vi "UserDIO and Binning Time to FPGA.vi"(8 "error in (no error)":errorcluster, 11 "FPGA VI Reference Out":refnum<k20>) -> (0 "error out":errorcluster)   [LabVIEW 2024]
uses:
  Type Definitions/DIO_Cluster.ctl
  <vilib>/Utility/error.llb/Error Cluster From Error Code.vi
  <vilib>/rvi/errors/niLvFpgaAdjustHostInterfaceError.vi
  <vilib>/rvi/interface/nirviReadWriteControl/nirviReadWriteControl.xnode
  NiFpgaLv.dll
  <vilib>/rvi/interface/Simulation/niFpgaSimulationCallBeginRW.vi
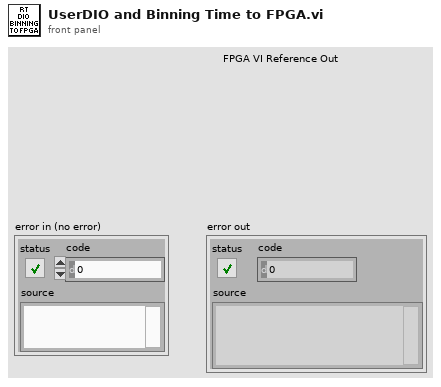
[diagram p1: front panel]
types:
  T1 = typedef "DIO_Cluster.ctl" = cluster{"DIO0":bool, "DIO1":bool, "DIO2":bool, "DIO3":bool}
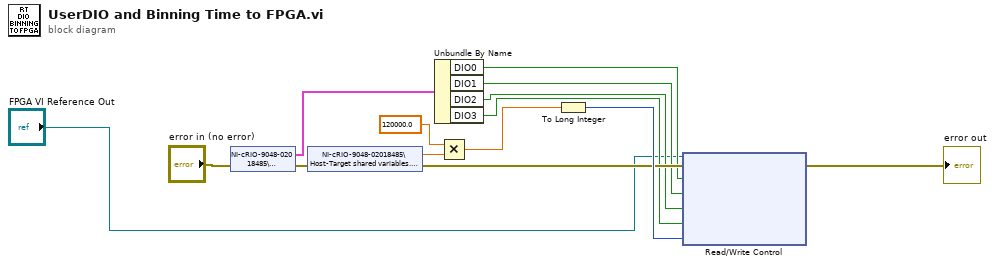
[diagram p0: block diagram]
diagram:
  n1 = shared-variable "NI-cRIO-9048-02018485\\Host-Target shared variables.lvlib\\DIO"(error in="error in (no error)") -> (w2:T1, error out=w8:errorcluster)
  n2 = shared-variable "NI-cRIO-9048-02018485\\Host-Target shared variables.lvlib\\Binning Time"(error in=w8) -> (w10:dbl, error out=w9:errorcluster)
  n3 = Unbundle By Name(w2) -> ("DIO0"=w4:bool, "DIO1"=w5:bool, "DIO2"=w6:bool, "DIO3"=w7:bool)
  n4 = Multiply(x=120000.0, y=w10) -> (x*y=w12:dbl)
  n5 = To Long Integer(number=w12) -> (32bit integer=w13:i32)
  n6 = xnode "Read/Write Control"("FPGA VI Reference In"="FPGA VI Reference Out", "error in"=w9, "DIO0"=w4, "DIO1"=w5, "DIO2"=w6, "DIO3"=w7, "Binning Time (ticks)"=w13) -> ("error out"=→"error out":errorcluster)  [unwired: 1 out]
